vi "Determine Cell Size and Position.vi"(8 "error in (no error)":errorcluster, 10 "Cell Position":T3, 11 "DataGrid in":refnum<class "DataGrid.lvclass">) -> (0 "error out":errorcluster, 1 "Properties:Active Cell Cell Size":T2, 2 "ScreenCoords":T1, 3 "DataGrid out":refnum<class "DataGrid.lvclass">)   [LabVIEW 2017, in "DataGrid.lvclass"]
uses:
  DataGrid.lvclass
  <vilib>/Utility/miscctls.llb/LVRowAndColumnTypeDef.ctl
  C:/Program Files (x86)/National Instruments/LabVIEW 2017/vi.lib/QSI/QControls/QControl Classes/MulticolumnListbox/MulticolumnListbox.lvclass
  C:/Program Files (x86)/National Instruments/LabVIEW 2017/vi.lib/QSI/QControls/QControl Classes/Generic/Generic.lvclass
  C:/Program Files (x86)/National Instruments/LabVIEW 2017/vi.lib/QSI/QControls/QControl Classes/Control/Control.lvclass
  <vilib>/Utility/miscctls.llb/LVBoundsTypeDef.ctl
  <vilib>/Utility/miscctls.llb/LVPointTypeDef.ctl
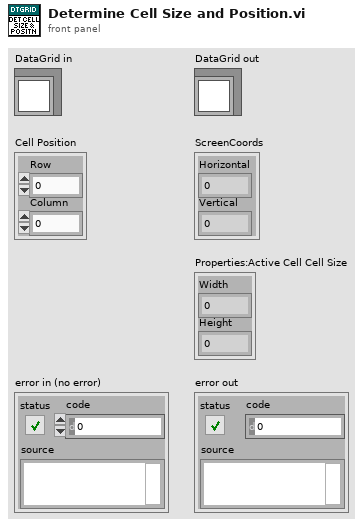
[diagram p1: front panel]
types:
  T1 = typedef "LVPointTypeDef.ctl" = cluster{"Horizontal":i16, "Vertical":i16}
  T2 = typedef "LVBoundsTypeDef.ctl" = cluster{"Width":u32, "Height":u32}
  T3 = typedef "LVRowAndColumnTypeDef.ctl" = cluster{"Row":i32, "Column":i32}
  T4 = typedef "LVPositionTypeDef.ctl" = cluster{"Left":i32, "Top":i32}
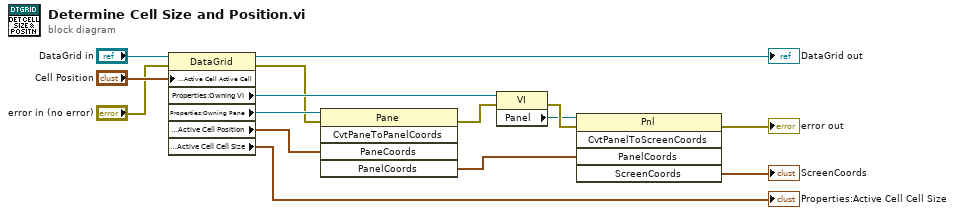
[diagram p0: block diagram]
diagram:
  n1 = property class="DataGrid"(reference="DataGrid in", error in="error in (no error)", "Properties:Active Cell Active Cell"="Cell Position") -> (reference out=→"DataGrid out":refnum<class "DataGrid.lvclass">, error out=w1:errorcluster, "Properties:Owning VI"=w5:refnum<vi>, "Properties:Owning Pane"=w3:refnum<vi>, "Properties:Active Cell Position"=w4:T4, "Properties:Active Cell Cell Size"=→"Properties:Active Cell Cell Size":T2)
  n2 = invoke class="Pane" method="CvtPaneToPanelCoords"(reference=w3, error in=w1, "PaneCoords"=w4) -> (error out=w6:errorcluster, "PanelCoords"=w8:T1)  [unwired: 2 in, 3 out]
  n3 = property class="VI"(reference=w5, error in=w6) -> (error out=w11:errorcluster, "Panel"=w7:refnum<vi>)  [unwired: 1 out]
  n4 = invoke class="Pnl" method="CvtPanelToScreenCoords"(reference=w7, error in=w11, "PanelCoords"=w8) -> (error out=→"error out":errorcluster, "ScreenCoords"=→"ScreenCoords":T1)  [unwired: 2 in, 3 out]
